vi "Write Name.vi"(8 "error in (no error)":errorcluster, 10 "Name":string, 11 "BaseReader in":refnum<class "BaseReader.lvclass">) -> (0 "error out":errorcluster, 3 "BaseReader out":refnum<class "BaseReader.lvclass">)   [LabVIEW 2013, in "BaseReader.lvclass"]
doc: "Sets the name of the reader"
uses:
  BaseReader.lvclass
  BaseReader.lvclass/BaseReader.ctl
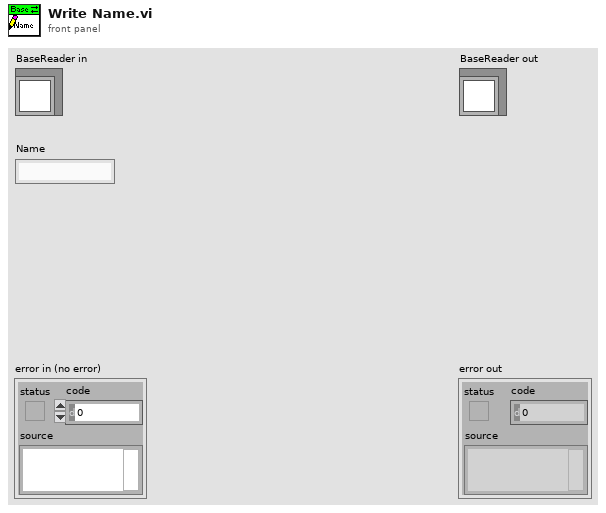
[diagram p1: front panel]
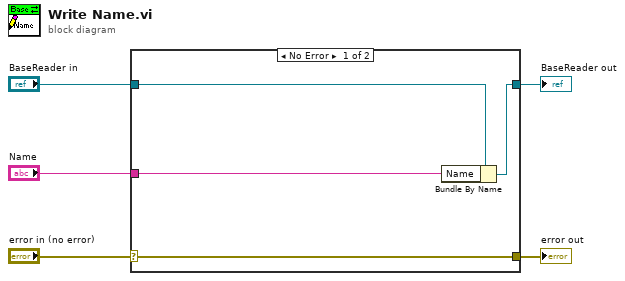
[diagram p0: block diagram]
diagram:
  n1 = case shown="No Error" "error in (no error)" {
    selector: "error in (no error)" -> [w9 w10]
    tunnel: [w9 w10] -> w4
    tunnel: [w7 w11] -> w2
    tunnel: "BaseReader in" -> [w8 w11]
    tunnel: "Name" -> [w6 _]
    frame No Error {
      n2 = Bundle By Name(cluster=w8, "Name"=w6) -> (w7:refnum<class "BaseReader.lvclass">)
    }
    frame Error {
    }
  }
  "error out" <- w4
  "BaseReader out" <- w2
